vi "Configure.vi"(0 "SG Path Power Meter Accessor in":refnum<class "SG Path Simulated PM Accessor.lvclass">, 5 "frequency":dbl=50000000.0, 11 "error in":errorcluster) -> (4 "SG Path Power Meter Accessor out":refnum<class "SG Path Simulated PM Accessor.lvclass">, 15 "error out":errorcluster)   [LabVIEW 2023, in "RFFixtureCharact.Instruments.lvlib" / "SG Path Simulated PM Accessor.lvclass"]
uses:
  SG Path Simulated PM Accessor.lvclass
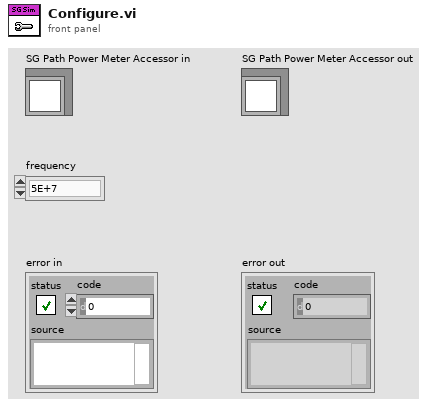
[diagram p1: front panel]
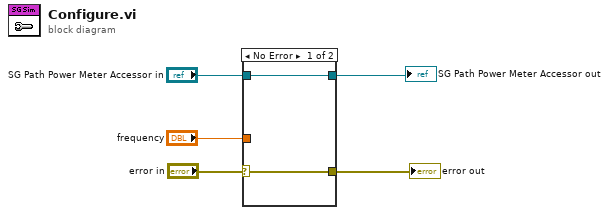
[diagram p0: block diagram]
diagram:
  n1 = case shown="No Error" "error in" {
    selector: "error in" -> [w7 w8]
    tunnel: [w7 w8] -> w1
    tunnel: [w6 w9] -> w4
    tunnel: "SG Path Power Meter Accessor in" -> [w6 w9]
    tunnel: "frequency" -> [_ _]
    frame No Error {
    }
    frame Error {
    }
  }
  "error out" <- w1
  "SG Path Power Meter Accessor out" <- w4
